vi "create_test_log_folder.vi"(8 "error in (no error)":errorcluster, 10 "values in":T1, 11 "config_file_name":string="config.ini") -> (0 "error out":errorcluster, 2 "values out":T1, 3 "config_file_name_out":string)   [LabVIEW 2015]
uses:
  Type Definitions/create_test_log_folder_states.ctl
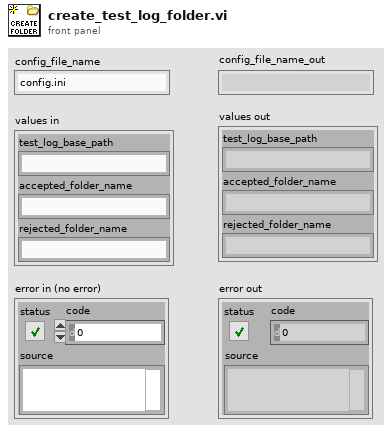
[diagram p1: front panel]
types:
  T1 = cluster{"test_log_base_path":string, "accepted_folder_name":string, "rejected_folder_name":string}
  T2 = typedef "create_test_log_folder_states.ctl" = enum16{"Initialize", "Create Test Log folder", "Create Accepted folder", "Create Rejected folder", "Shutdown"}
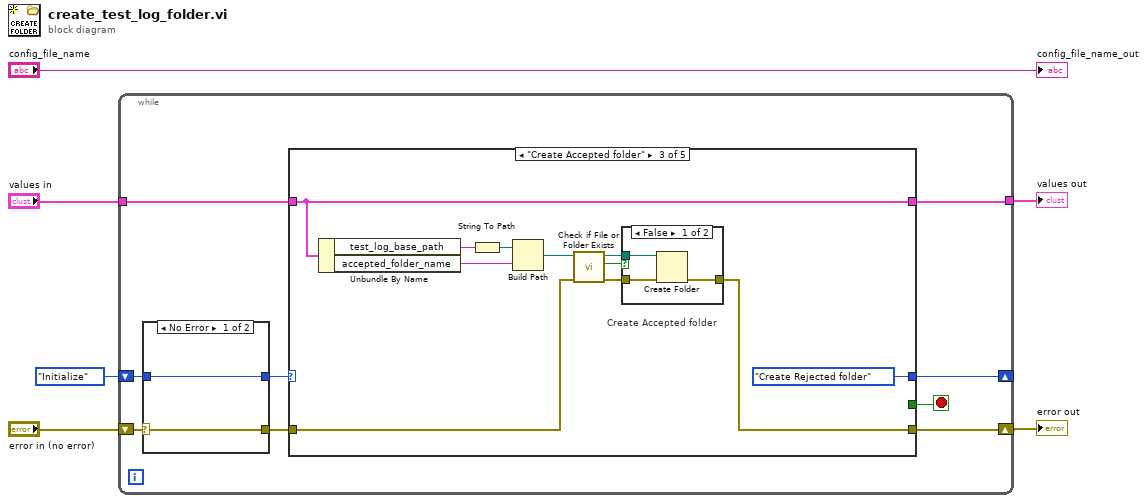
[diagram p0: block diagram]
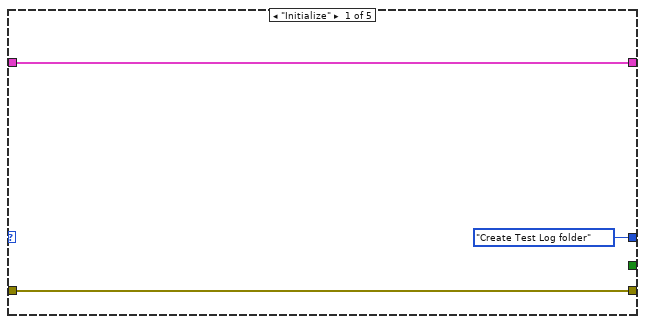
[diagram p2: hidden frame]
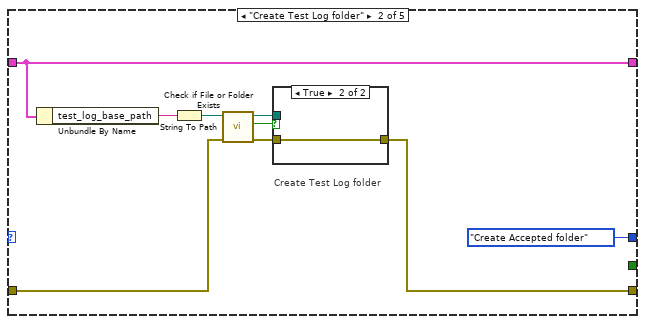
[diagram p3: hidden frame]
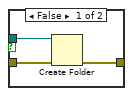
[diagram p4: hidden frame]
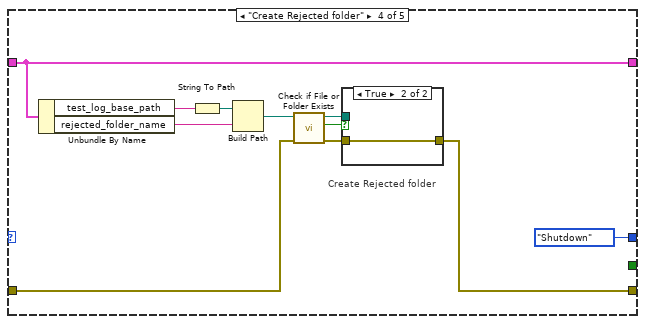
[diagram p6: hidden frame]
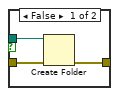
[diagram p7: hidden frame]
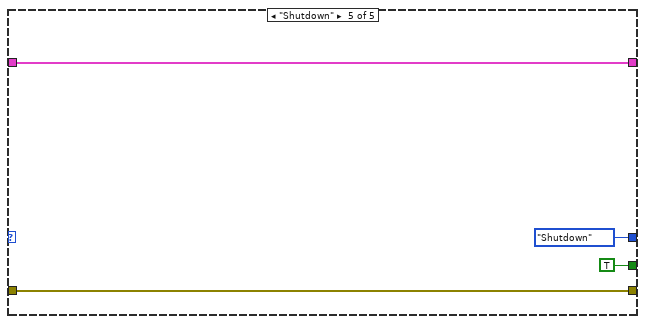
[diagram p8: hidden frame]
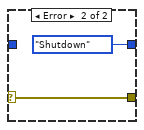
[diagram p9: hidden frame]
diagram:
  n1 = while {
    shift-right: [w13] -> w3
    shift-left: "error in (no error)" -> [w15]
    shift-right: [w10] -> _
    shift-left: create_test_log_folder_states."Initialize" -> [w12]
    tunnel: "values in" -> [w8]
    tunnel: [w7] -> w1
    stop <- w9 stop-if-true
    n2 = case shown="No Error" w15 {
      selector: w15 -> [w66 w69]
      tunnel: [w66 w69] -> w14
      tunnel: w12 -> [w67 _]
      tunnel: [w67 create_test_log_folder_states."Shutdown"] -> w11
      frame No Error {
      }
      frame Error {
      }
    }
    n3 = case shown="\"Create Accepted folder\"" w11 {
      tunnel: w14 -> [w18 w24 w36 w50 w63]
      tunnel: [w18 w23 w35 w47 w63] -> w13
      tunnel: [create_test_log_folder_states."Create Test Log folder" create_test_log_folder_states."Create Accepted folder" create_test_log_folder_states."Create Rejected folder" create_test_log_folder_states."Shutdown" create_test_log_folder_states."Shutdown"] -> w10
      tunnel: [_ _ _ _ TRUE] -> w9
      tunnel: w8 -> [w16 w19 w32 w51 w62]
      tunnel: [w16 w19 w32 w51 w62] -> w7
      frame "Initialize" {
      }
      frame "Create Test Log folder" {
        # "Create Test Log folder"
        n4 = Unbundle By Name(w19) -> ("test_log_base_path"=w22:string)
        n5 = String To Path(string=w22) -> (path=w21:path)
        n6 = call <vilib>:"Check if File or Folder Exists.vi"("error in (no error)"=w24, "path"=w21) -> ("error out"=w27:errorcluster, "file or folder exists?"=w25:bool, "dup path"=w26:path)  [unwired: 7 in]
        n7 = case shown="True" w25 {
          tunnel: w26 -> [w30 _]
          tunnel: w27 -> [w29 w31]
          tunnel: [w28 w31] -> w23
          frame False {
            n8 = Create Folder(path (use dialog)=w30, error in=w29) -> (error out=w28:errorcluster)  [unwired: 1 in, 2 out]
          }
          frame True {
          }
        }
      }
      frame "Create Accepted folder" {
        # "Create Accepted folder"
        n9 = Unbundle By Name(w32) -> ("test_log_base_path"=w40:string, "accepted_folder_name"=w39:string)
        n10 = String To Path(string=w40) -> (path=w41:path)
        n11 = Build Path(base path=w41, name or relative path=w39) -> (appended path=w38:path)
        n12 = call <vilib>:"Check if File or Folder Exists.vi"("error in (no error)"=w36, "path"=w38) -> ("error out"=w42:errorcluster, "file or folder exists?"=w33:bool, "dup path"=w37:path)  [unwired: 7 in]
        n13 = case shown="False" w33 {
          tunnel: w37 -> [w45 _]
          tunnel: w42 -> [w44 w46]
          tunnel: [w43 w46] -> w35
          frame False {
            n14 = Create Folder(path (use dialog)=w45, error in=w44) -> (error out=w43:errorcluster)  [unwired: 1 in, 2 out]
          }
          frame True {
          }
        }
      }
      frame "Create Rejected folder" {
        # "Create Rejected folder"
        n15 = Unbundle By Name(w51) -> ("test_log_base_path"=w55:string, "rejected_folder_name"=w54:string)
        n16 = String To Path(string=w55) -> (path=w56:path)
        n17 = Build Path(base path=w56, name or relative path=w54) -> (appended path=w53:path)
        n18 = call <vilib>:"Check if File or Folder Exists.vi"("error in (no error)"=w50, "path"=w53) -> ("error out"=w57:errorcluster, "file or folder exists?"=w48:bool, "dup path"=w52:path)  [unwired: 7 in]
        n19 = case shown="True" w48 {
          tunnel: w52 -> [w60 _]
          tunnel: w57 -> [w59 w61]
          tunnel: [w58 w61] -> w47
          frame False {
            n20 = Create Folder(path (use dialog)=w60, error in=w59) -> (error out=w58:errorcluster)  [unwired: 1 in, 2 out]
          }
          frame True {
          }
        }
      }
      frame "Shutdown" {
      }
    }
  }
  "error out" <- w3
  "values out" <- w1
  "config_file_name_out" <- "config_file_name"
